vi "SendData.vi"(8 "error in (no error)":errorcluster, 9 "Length of \nData bundle":i32, 10 "SerialisedData":string, 11 "DataPacker in":refnum<class "DataPacker.lvclass">) -> (0 "error out":errorcluster, 2 "MIDAS Reply":string, 3 "DataPacker out":refnum<class "DataPacker.lvclass">)   [LabVIEW 2018, in "feGEM DataPacker.lvlib"]
uses:
  feGEM DataPacker.lvlib
  DataPacker.lvclass
  GlobalVariables/Set_And_Get_Enum.ctl
  <vilib>/Utility/SystemLogging/NI_SystemLogging.lvlib
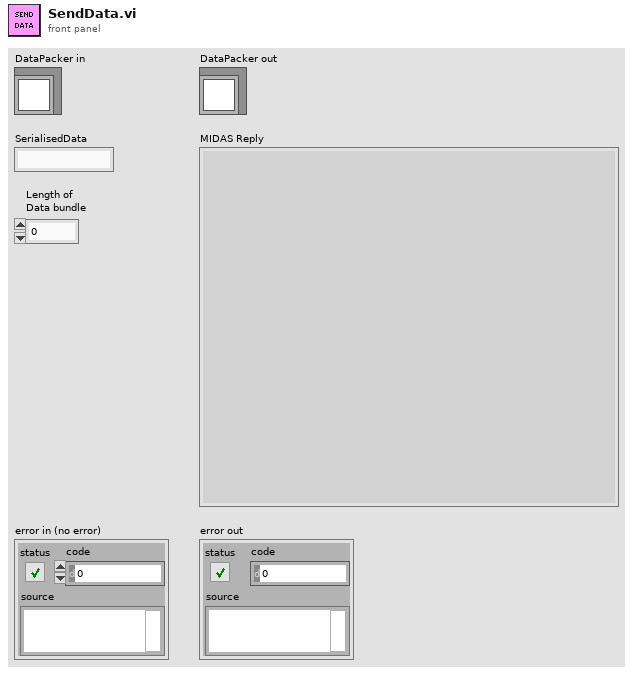
[diagram p1: front panel]
types:
  T1 = typedef "feGEM DataPacker.lvlib/Set_And_Get_Enum.ctl" = enum16{"Set", "Get"}
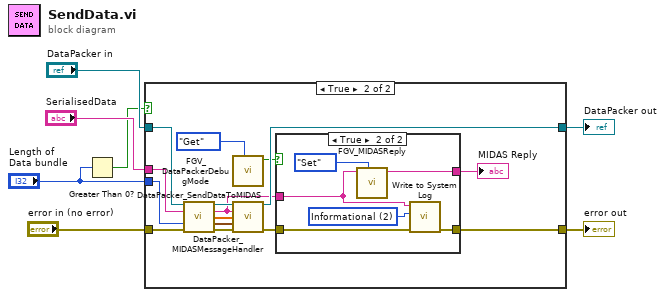
[diagram p0: block diagram]
diagram:
  n1 = Greater Than 0?(x="Length of \nData bundle") -> (x > 0?=w1:bool)
  n2 = case shown="True" w1 {
    tunnel: "Length of \nData bundle" -> [_ w18]
    tunnel: "SerialisedData" -> [_ w22]
    tunnel: "DataPacker in" -> [w9 w20]
    tunnel: "error in (no error)" -> [w8 w19]
    tunnel: [w8 w13] -> w5
    tunnel: [w9 w21] -> w4
    frame False {
    }
    frame True {
      n3 = call "DataPacker_SendDataToMIDAS.vi"("DataPacker in"=w20, "data in"=w22, "data in length"=w18, "error in (no error)"=w19) -> ("DataPacker out"=w23:refnum<class "DataPacker.lvclass">, "MIDAS Reply"=w15:string, "Send Time, Recieve Time"=w16:dbl[], "MIDAS Comm finished"=w17:timestamp, "error out"=w24:errorcluster)  [unwired: 7 in]
      n4 = call "FGV_DataPackerDebugMode.vi"(7:Set_And_Get_Enum."Get") -> ("Debug Mode"=w12:bool)  [unwired: 10 in]
      n5 = call "DataPacker_MIDASMessageHandler.vi"("DataPacker in"=w23, "Message"=w15, "Array"=w16, "MIDAS Comm finish time"=w17, "error in (no error)"=w24) -> ("DataPacker out"=w21:refnum<class "DataPacker.lvclass">, "error out"=w14:errorcluster)  [unwired: 9 in]
      n6 = case shown="True" w12 {
        tunnel: w15 -> [w25 w28]
        tunnel: w14 -> [w26 w31]
        tunnel: [w26 w30] -> w13
        tunnel: [w25 w27] -> w10
        frame False {
        }
        frame True {
          w32 = 2 items=["Error", "Warning", "Informational"] ("severity")
          n7 = call "FGV_MIDASReply.vi"("Enum"=Set_And_Get_Enum."Set", "MIDAS Reply"=w28) -> ("MIDAS Reply"=w27:string)  [unwired: 9 in]
          n8 = call <vilib>:"Write to System Log.vi"("error in (no error)"=w31, "severity"=w32, "message"=w28) -> ("error out"=w30:errorcluster)  [unwired: 8 in]
        }
      }
      "MIDAS Reply" <- w10
    }
  }
  "error out" <- w5
  "DataPacker out" <- w4
